vi "Upload Package to SystemLink Repository.vi"(0 "SystemLink repo in":T1, 5 "package filepath":path, 9 "timeout (ms) (10000)":u32=10000, 11 "error in (no error)":errorcluster) -> (4 "SystemLink repo out":T1, 8 "package ID":string, 10 "timed out?":bool, 15 "error out":errorcluster)   [LabVIEW 2017, in "SystemLink_Repo_API.lvlib"]
doc: "Uploads the package to the SystemLink repository and waits until the specified job returns a status of \"succeeded\" or \"failed\".\n\nInputs:\nPackage filepath - This is the filepath of the package (.nipkg, .ipk) you want to upload.\n\nOutputs:\nPackage ID - Returns the package ID in the SystemLink repository that corresponds to the uploaded package file.\n\nError Handling:\nOutputs Error 6000 if the upload job fails.\nOutputs Error 6001 if the upload job does not return a status of \"succeeded\" or \"failed\" within the timeout period."
uses:
  SystemLink_Repo_API.lvlib
  <vilib>/httpClient/ClientHandle.ctl
  <vilib>/httpClient/LabVIEWHTTPClient.lvlib
  _support/systemlink repo.ctl
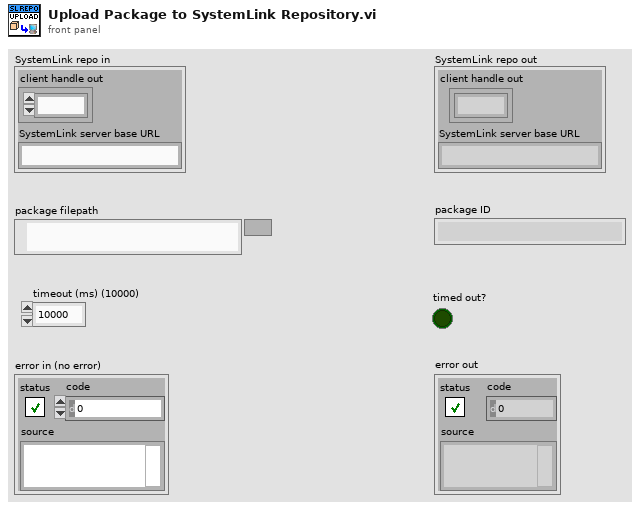
[diagram p1: front panel]
types:
  T1 = typedef "SystemLink_Repo_API.lvlib/systemlink repo.ctl" = cluster{"client handle out":T2, "SystemLink server base URL":string}
  T2 = typedef "LabVIEWHTTPClient.lvlib/ClientHandle.ctl" = refnum<k1>
  T3 = typedef "SystemLink_Repo_API.lvlib/syslink_job.ctl" = cluster{"job":T4}
  T4 = typedef "SystemLink_Repo_API.lvlib/syslink_job_datatype.ctl" = cluster{"id":string, "operation":string, "status":string, "error":cluster{"name":string, "message":string, "args":string[], "innerErrors":string[]}, "created":string, "resourceId":string, "resourceIds":string[], "returnType":string}
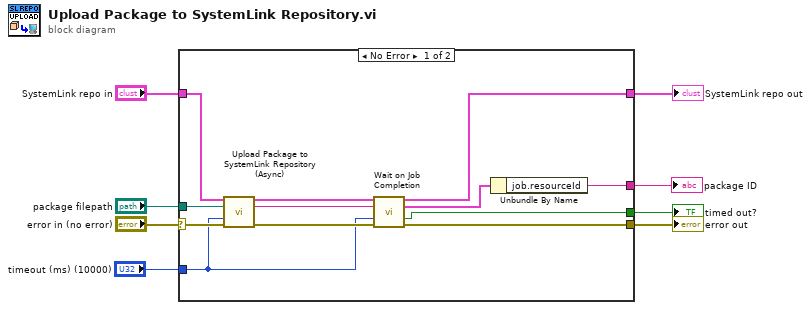
[diagram p0: block diagram]
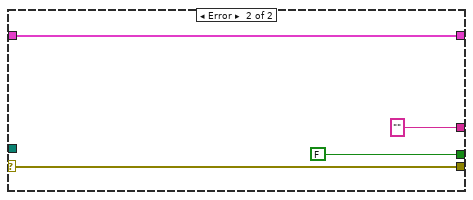
[diagram p2: hidden frame]
diagram:
  n1 = case shown="No Error" "error in (no error)" {
    selector: "error in (no error)" -> [w20 w24]
    tunnel: "SystemLink repo in" -> [w15 w23]
    tunnel: [w13 w24] -> w6
    tunnel: "package filepath" -> [w19 _]
    tunnel: [w14 w23] -> w4
    tunnel: "timeout (ms) (10000)" -> [w9 _]
    tunnel: [w10 FALSE ("timed out?")] -> w2
    tunnel: [w11 "" ("resourceId")] -> w1
    frame No Error {
      n2 = call "Upload Package to SystemLink Repository (Async).vi"("SystemLink repo in"=w15, "package filepath"=w19, "timeout (ms) (10000)"=w9, "error in (no error)"=w20) -> ("SystemLink repo out"=w17:T1, "jobID"=w16:string, "error out"=w18:errorcluster)  [unwired: 9 in]
      n3 = call "Wait on Job Completion.vi"("SystemLink repo in"=w17, "job ID"=w16, "timeout (ms) (10000)"=w9, "error in (no error)"=w18) -> ("SystemLink repo out"=w14:T1, "job data"=w12:T3, "timed out?"=w10:bool, "error out"=w13:errorcluster)  [unwired: 8 in]
      n4 = Unbundle By Name(w12) -> ("job.resourceId"=w11:string)
    }
    frame Error {
    }
  }
  "error out" <- w6
  "SystemLink repo out" <- w4
  "timed out?" <- w2
  "package ID" <- w1
